vi "Between.vi"() -> ()   [LabVIEW 2014]
panel:
  in  "Gap":dbl
  in  "Edge":dbl
  in  "Shape":bool
  in  "n by n":dbl
  out "Spinning Angle":string
  out "Number":string
  in  "Between Series":dbl=2.0
  in  "Between Pattern":dbl=0.5
  in  "Pattern":string(combo)="Gradient"
  in  "Radius":i32=120
  in  "Angle":string(combo)="0"
  in  "Start":bool
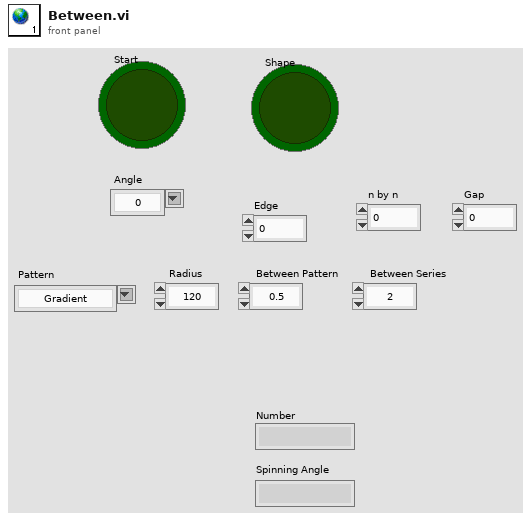
[diagram p1: front panel]
diagram:
